vi "Subtract Rational Polynomials (CDB).vi"(4 "threshold type":T1 items=["Absolute Value", "Relative Value"], 6 "threshold":dbl, 8 "Denominator 2":cdb[](array[numeric]) format="%#.2g", 9 "Numerator 2":cdb[](array[numeric]) format="%#.2g", 10 "Denominator 1":cdb[](array[numeric]) format="%#.2g", 11 "Numerator 1":cdb[](array[numeric]) format="%#.2g") -> (0 "error":i32, 2 "Denominator Out":cdb[](array[numeric]) format="%#.2g", 3 "Numerator Out":cdb[](array[numeric]) format="%#.2g")   [LabVIEW 2014, in "NI_AALPro.lvlib"]
doc: "Subtracts rational polynomial G2 from rational polynomial G1. The data types you wire to the <B>Numerator 1</B>, <B>Denominator 1</B>, <B>Numerator 2</B>, and <B>Denominator 2</B> inputs determine the polymorphic instance to use."
uses:
  NI_AALPro.lvlib
  Remove Zero Threshold Type.ctl
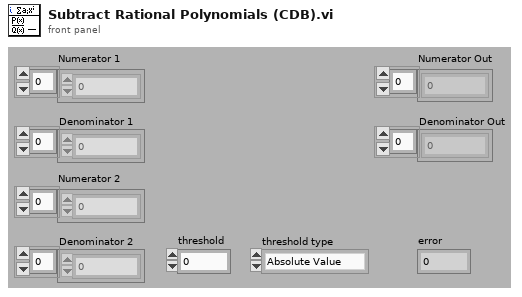
[diagram p1: front panel]
types:
  T1 = typedef "NI_AALPro.lvlib/Remove Zero Threshold Type.ctl" = u16
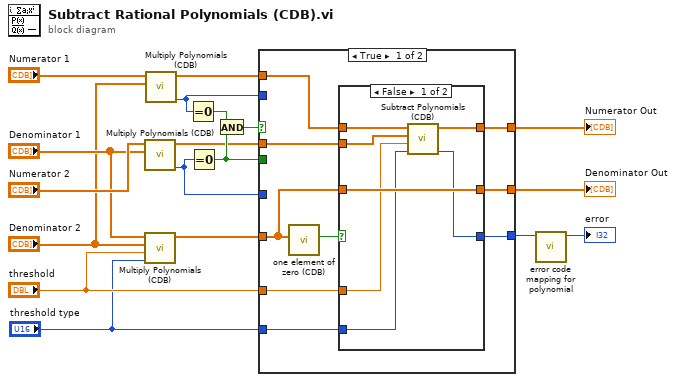
[diagram p0: block diagram]
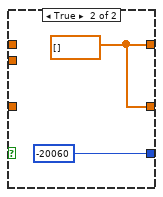
[diagram p2: hidden frame]
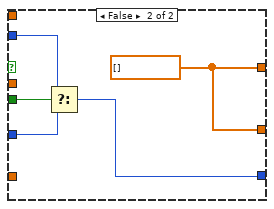
[diagram p3: hidden frame]
diagram:
  n1 = call "Multiply Polynomials (CDB).vi"("Q(x)"="Denominator 1", "P(x)"="Numerator 2") -> ("error"=w3:i32, "P(x)*Q(x)"=w4:cdb[])  [unwired: 8 in]
  n2 = call "Multiply Polynomials (CDB).vi"("threshold type"="threshold type", "threshold"="threshold", "Q(x)"="Denominator 2", "P(x)"="Denominator 1") -> ("P(x)*Q(x)"=w5:cdb[])  [unwired: 6 in, 1 out]
  n3 = call "Multiply Polynomials (CDB).vi"("Q(x)"="Denominator 2", "P(x)"="Numerator 1") -> ("error"=w9:i32, "P(x)*Q(x)"=w10:cdb[])  [unwired: 8 in]
  n4 = Equal To 0?(x=w9) -> (x = 0?=w14:bool)
  n5 = Equal To 0?(x=w3) -> (x = 0?=w12:bool)
  n6 = And(x=w14, y=w12) -> (x .and. y?=w13:bool)
  n7 = case shown="True" w13 {
    tunnel: w10 -> [w27 _]
    tunnel: w4 -> [w26 _]
    tunnel: [w25 w41] -> w18
    tunnel: w5 -> [w24 _]
    tunnel: [w22 w41] -> w17
    tunnel: [w21 w37] -> w16
    tunnel: w9 -> [_ w38]
    tunnel: w3 -> [_ w39]
    tunnel: w12 -> [_ w40]
    tunnel: "threshold" -> [w20 _]
    tunnel: "threshold type" -> [w19 _]
    frame True {
      n8 = call "one element of zero (CDB).vi"("Array in"=w24) -> ("equal [0]?"=w23:bool)  [unwired: 10 in]
      n9 = case shown="False" w23 {
        tunnel: w27 -> [w34 _]
        tunnel: w26 -> [w33 _]
        tunnel: [w31 w36] -> w25
        tunnel: w24 -> [w32 _]
        tunnel: [w32 w36] -> w22
        tunnel: [w30 -20060 ("divide by zero")] -> w21
        tunnel: w20 -> [w29 _]
        tunnel: w19 -> [w28 _]
        frame False {
          n10 = call "Subtract Polynomials (CDB).vi"("threshold type"=w28, "threshold"=w29, "Q(x)"=w33, "P(x)"=w34) -> ("error"=w30:i32, "P(x)-Q(x)"=w31:cdb[])  [unwired: 6 in]
        }
        frame True {
          w36 = cdb[] [] ("CDB")
        }
      }
    }
    frame False {
      w41 = cdb[] [] ("CDB")
      n11 = Select(t=w38, s=w40, f=w39) -> (s? t:f=w37:i32)
    }
  }
  "Numerator Out" <- w18
  "Denominator Out" <- w17
  n12 = call "error code mapping for polynomial.vi"("error in"=w16) -> ("error out"=→"error":i32)  [unwired: 10 in]
